vi "Ist mit Soll vergleichen Regler.vi"(8 "error in (no error)":errorcluster caption="Fehler (Eingang, kein Fehler)", 10 "Index":u16, 11 "Schneider Steuerung PNS Eingang":refnum<class "Schneider Steuerung PNS.lvclass">) -> (0 "error out":errorcluster caption="Fehler (Ausgang)", 2 "Werte":cluster{u16[], u16[]}, 3 "Schneider Steuerung PNS Ausgang":refnum<class "Schneider Steuerung PNS.lvclass">)   [LabVIEW 2020, in "Schneider Steuerung PNS.lvclass"]
uses:
  Schneider Steuerung PNS.lvclass
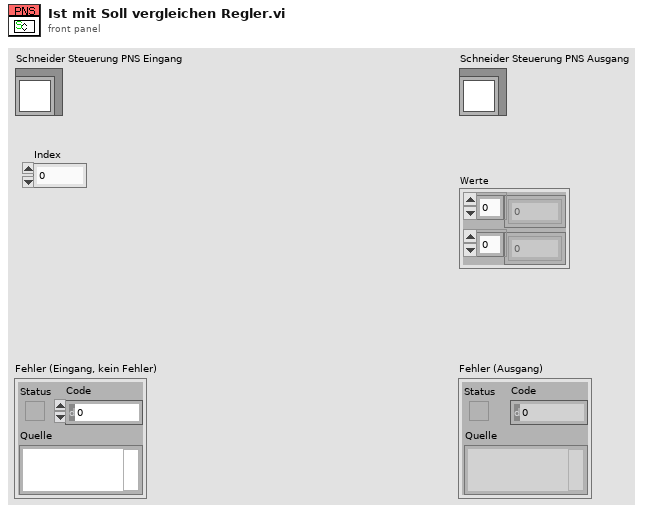
[diagram p1: front panel]
types:
  T1 = typedef "Steuerung PNS.lvclass/Anlegengrenzwerte PNS.ctl" = cluster{"Filter:":T2, "Ventilplatte:":T2, "Heizleitung 1:":T2, "Heizleitung 2:":T2, "Heizleitung 3:":T2, "Heizleitung 4:":T2, "Heizleitung 5:":T2, "Heizleitung 6:":T2}
  T2 = typedef "Steuerung PNS.lvclass/Anlagengrenzwerte Parameteranzeige.ctl" = cluster{"Sollwert":T3, "Warn-Min":T3, "Warn-Max":T3, "Abschalt-Min":T3, "Abschalt-Max":T3, "Regler":u16, "AnlagenParameter":string}
  T3 = typedef "Zahlen-Eingabefeld.ctl" = sgl
  T4 = typedef "Steuerung PNS.lvclass/Regler.ctl" = cluster{"Istwert":i16, "Sollwert":i16, "Alarm MIN":i16, "Alarm MAX":i16, "Regler sperren":i16, "Analog Ausgang":i16}[]
  T5 = cluster{"Istwert":i16, "Sollwert":i16, "Alarm MIN":i16, "Alarm MAX":i16, "Regler sperren":i16, "Analog Ausgang":i16}
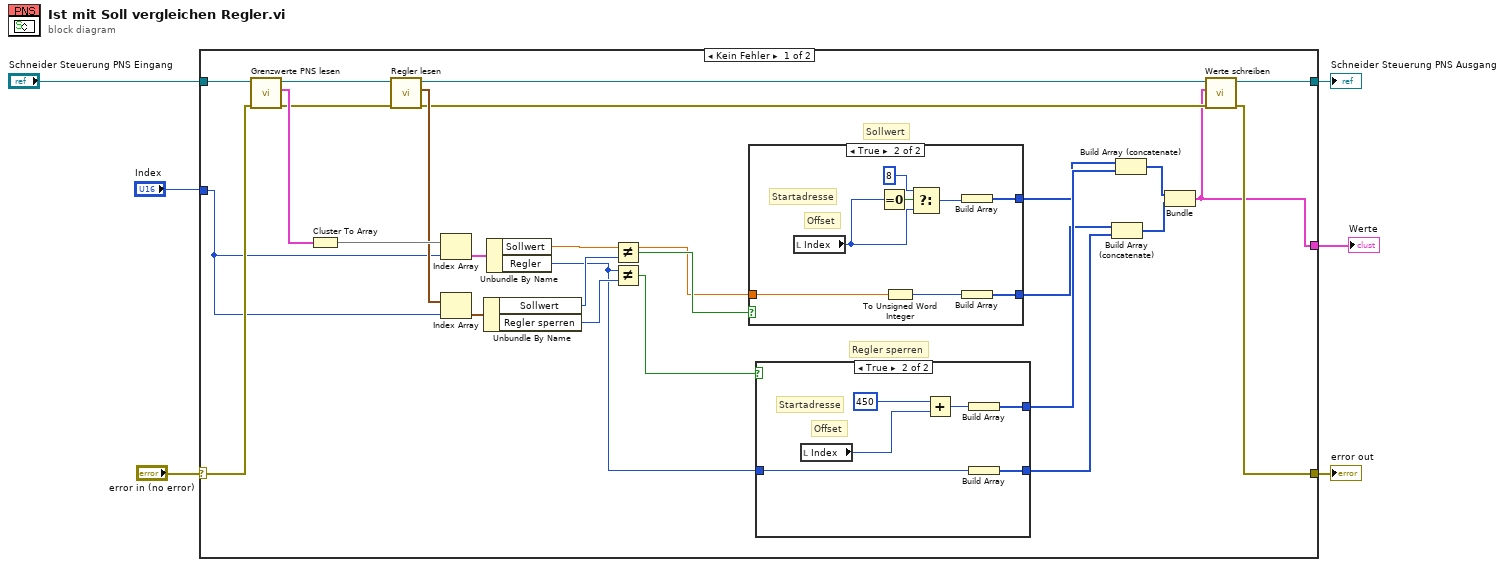
[diagram p0: block diagram]
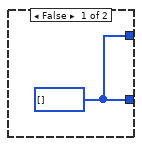
[diagram p2: hidden frame]
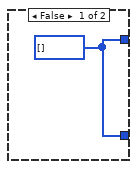
[diagram p3: hidden frame]
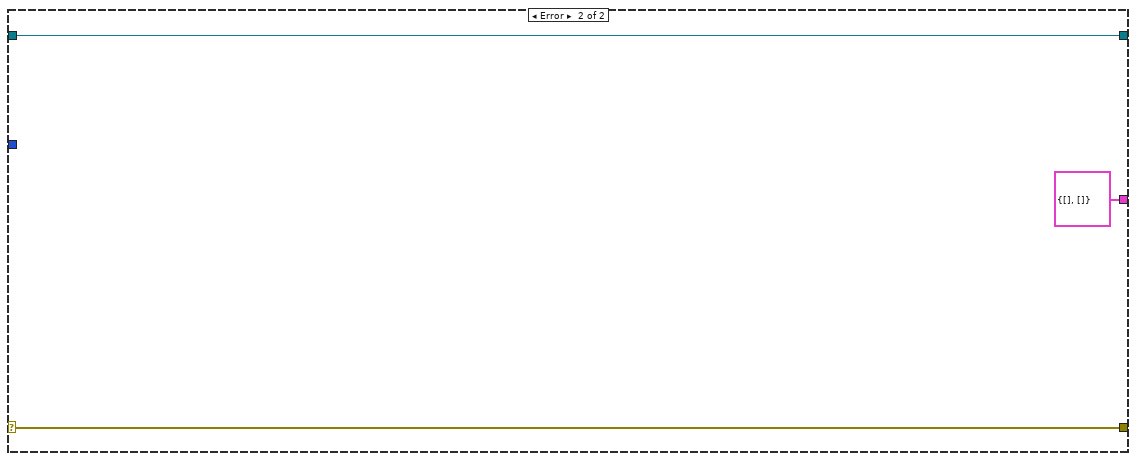
[diagram p4: hidden frame]
diagram:
  n1 = case shown="Kein Fehler" "error in (no error)" {
    selector: "error in (no error)" -> [w12 w52]
    tunnel: [w11 w52] -> w5
    tunnel: [w15 w51] -> w3
    tunnel: "Schneider Steuerung PNS Eingang" -> [w16 w51]
    tunnel: "Index" -> [w7 _]
    tunnel: [w8 cluster{u16[], u16[]} {[], []}] -> w1
    frame No Error {
      # "Regler sperren"
      # "Sollwert"
      n2 = call-dynamic "Grenzwerte PNS lesen.vi"("error in (no error)"=w12, "Steuerung PNS (Eingang)"=w16) -> ("error out"=w13:errorcluster, "Grenzwerte PNS"=w20:T1, "Steuerung PNS (Ausgang)"=w10:refnum<class "Schneider Steuerung PNS.lvclass">)  [unwired: 7 in]
      n3 = Cluster To Array(cluster=w20) -> (array=w33:T2[])
      n4 = call-dynamic "Regler lesen.vi"("error in (no error)"=w13, "Steuerung PNS (Eingang)"=w10) -> ("error out"=w14:errorcluster, "Regler"=w19:T4, "Steuerung PNS (Ausgang)"=w9:refnum<class "Schneider Steuerung PNS.lvclass">)  [unwired: 7 in]
      n5 = Index Array(array=w33, index=w7) -> (element=w32:T2)
      n6 = Index Array(array=w19, index=w7) -> (element=w31:T5)
      n7 = Unbundle By Name(w31) -> ("Sollwert"=w30:i16, "Regler sperren"=w29:i16)
      n8 = Unbundle By Name(w32) -> ("Sollwert"=w27:T3, "Regler"=w26:u16)
      n9 = Not Equal?(x=w27, y=w30) -> (x != y?=w28:bool)
      n10 = Not Equal?(x=w26, y=w29) -> (x != y?=w25:bool)
      n11 = case shown="True" w28 {
        tunnel: w27 -> [_ w49]
        tunnel: [w41 w47] -> w22
        tunnel: [w41 w46] -> w21
        frame False {
          w41 = u16[] []
        }
        frame True {
          # "Offset"
          # "Startadresse"
          n12 = local read "Index"() -> (w42:u16)
          n13 = Equal To 0?(x=w42) -> (x = 0?=w45:bool)
          n14 = To Unsigned Word Integer(number=w49) -> (unsigned 16bit integer=w48:u16)
          n15 = Select(t=u16 8, s=w45, f=w42) -> (s? t:f=w43:u16)
          n16 = Build Array(w43) -> (w47:u16[])
          n17 = Build Array(w48) -> (w46:u16[])
        }
      }
      n18 = case shown="True" w25 {
        tunnel: w26 -> [_ w36]
        tunnel: [w34 w38] -> w24
        tunnel: [w34 w37] -> w23
        frame False {
          w34 = u16[] []
        }
        frame True {
          # "Offset"
          # "Startadresse"
          n19 = local read "Index"() -> (w35:u16)
          n20 = Add(x=u16 450, y=w35) -> (x+y=w39:u16)
          n21 = Build Array(w39) -> (w38:u16[])
          n22 = Build Array(w36) -> (w37:u16[])
        }
      }
      n23 = Build Array (concatenate)(w21, w23) -> (w17:u16[])
      n24 = Build Array (concatenate)(w22, w24) -> (w18:u16[])
      n25 = Bundle(w18, w17) -> (w8:cluster{u16[], u16[]})  [unwired: 1 in]
      n26 = call-dynamic "Werte schreiben.vi"("error in (no error)"=w14, "Werte"=w8, "Steuerung PNS (Eingang)"=w9) -> ("error out"=w11:errorcluster, "Steuerung PNS (Ausgang)"=w15:refnum<class "Schneider Steuerung PNS.lvclass">)  [unwired: 7 in]
    }
    frame Error {
    }
  }
  "error out" <- w5
  "Schneider Steuerung PNS Ausgang" <- w3
  "Werte" <- w1
